vi "Align.vi"(6 "Variant in":variant, 7 "Shift Pressed?":bool, 8 "error in (no error)":errorcluster, 10 "QD Combo Box Ref":refnum<vi>, 11 "QD Launch VI Ref":refnum<vi>) -> (0 "error out":errorcluster, 4 "Variant out":variant)   [LabVIEW 2019]
doc: "Write a 1-2 sentence description of the functionality of your plugin here. Replace the \"$\" below with the character you wish to assign as the default shortcut for this plugin. Do not add any text after the 'Default Shortcut' line below.\n\nDefault Shortcut - [$]"
uses:
  <vilib>/Utility/traverseref.llb/TRef TravTarget.ctl
  <vilib>/Utility/traverseref.llb/VI Scripting - Traverse.lvlib
panel:
  in  "Undo Name":string="Quick Drop Keyboard Shortcut"
  # "Specify the name of the Undo transaction"
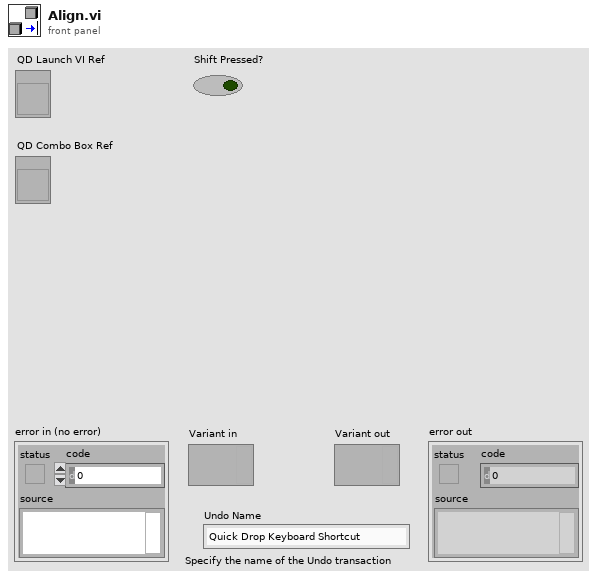
[diagram p1: front panel]
types:
  T1 = typedef "TRef TravTarget.ctl" = enum16{"FP", "BD", "Other"}
  T2 = enum32{"Top Edges", "Vertical Centers", "Bottom Edges", "Left Edges", "Horizontal Centers", "Right Edges"}
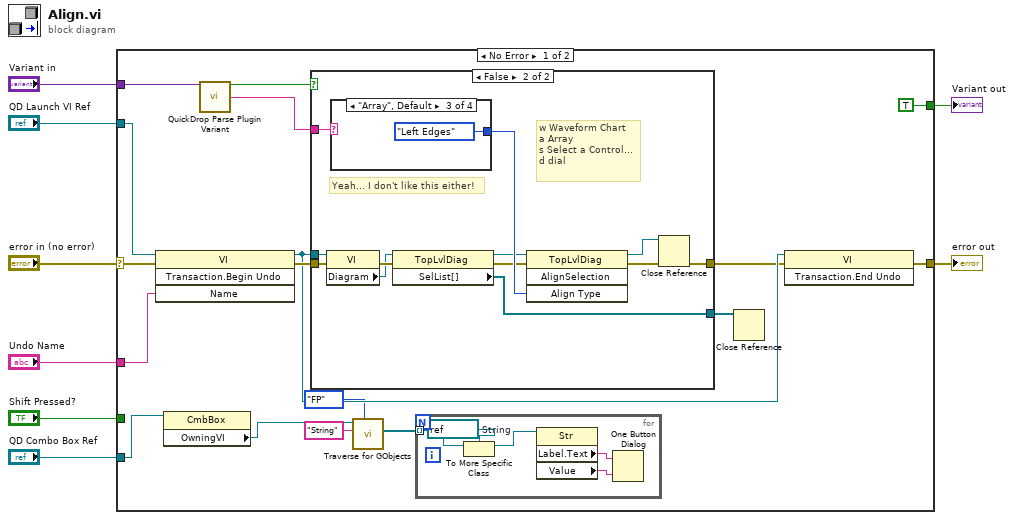
[diagram p0: block diagram]
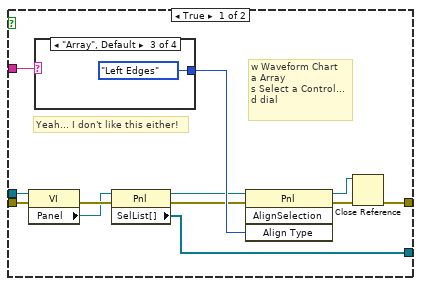
[diagram p2: hidden frame]
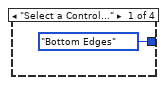
[diagram p3: hidden frame]
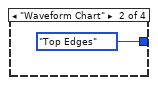
[diagram p4: hidden frame]
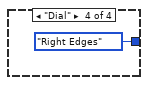
[diagram p5: hidden frame]
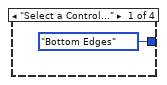
[diagram p6: hidden frame]
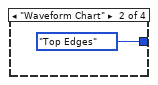
[diagram p7: hidden frame]
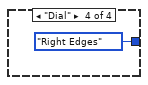
[diagram p8: hidden frame]
diagram:
  n1 = case shown="No Error" "error in (no error)" {
    selector: "error in (no error)" -> [w24 w63]
    tunnel: [w18 w63] -> w7
    tunnel: "QD Launch VI Ref" -> [w23 _]
    tunnel: "Shift Pressed?" -> [_ _]
    tunnel: "QD Combo Box Ref" -> [w13 _]
    tunnel: "Variant in" -> [w25 _]
    tunnel: "Undo Name" -> [w22 _]
    tunnel: [TRUE _] -> w1
    frame No Error {
      n2 = invoke class="VI" method="Transaction.Begin Undo"(reference=w23, error in=w24, "Name"=w22) -> (reference out=w17:refnum<vi>, error out=w19:errorcluster)  [unwired: 1 in, 2 out]
      n3 = property class="CmbBox"(reference=w13) -> ("OwningVI"=w12:refnum<vi>)  [unwired: 1 in, 2 out]
      n4 = call <vilib>:"QuickDrop Parse Plugin Variant.vi"("QDKS Variant in"=w25) -> ("QD Launch VI Panel?"=w20:bool, "Palette Object Name"=w16:string)  [unwired: 12 in, 1 out]
      n5 = case shown="False" w20 {
        tunnel: w19 -> [w42 w58]
        tunnel: w17 -> [w41 w57]
        tunnel: [w39 w47] -> w14
        tunnel: [w38 w55] -> w15
        tunnel: w16 -> [w35 w52]
        frame True {
          # "Yeah... I don't like this either!"
          # "w Waveform Chart\na Array\ns Select a Control...\nd dial"
          n6 = property class="VI"(reference=w41, error in=w42) -> (error out=w40:errorcluster, "Panel"=w37:refnum<vi>)  [unwired: 1 out]
          n7 = case shown="\"Array\", Default" w35 {
            tunnel: [T2."Bottom Edges" ("Align Type") T2."Top Edges" ("Align Type") T2."Left Edges" ("Align Type") T2."Right Edges" ("Align Type")] -> w36
            frame "Select a Control..." {
            }
            frame "Waveform Chart" {
            }
            frame "Array", Default {
            }
            frame "Dial" {
            }
          }
          n8 = property class="Pnl"(reference=w37, error in=w40) -> (reference out=w31:refnum<vi>, error out=w32:errorcluster, "SelList[]"=w38:refnum<vi>[])
          n9 = invoke class="Pnl" method="AlignSelection"(reference=w31, error in=w32, "Align Type"=w36) -> (reference out=w34:refnum<vi>, error out=w33:errorcluster)  [unwired: 1 in, 2 out]
          n10 = Close Reference(reference=w34, error in (no error)=w33) -> (error out=w39:errorcluster)
        }
        frame False {
          # "Yeah... I don't like this either!"
          # "w Waveform Chart\na Array\ns Select a Control...\nd dial"
          n11 = property class="VI"(reference=w57, error in=w58) -> (error out=w56:errorcluster, "Diagram"=w54:refnum<vi>)  [unwired: 1 out]
          n12 = case shown="\"Array\", Default" w52 {
            tunnel: [T2."Bottom Edges" ("Align Type") T2."Top Edges" ("Align Type") T2."Left Edges" ("Align Type") T2."Right Edges" ("Align Type")] -> w53
            frame "Select a Control..." {
            }
            frame "Waveform Chart" {
            }
            frame "Array", Default {
            }
            frame "Dial" {
            }
          }
          n13 = property class="TopLvlDiag"(reference=w54, error in=w56) -> (reference out=w51:refnum<vi>, error out=w50:errorcluster, "SelList[]"=w55:refnum<vi>[])
          n14 = invoke class="TopLvlDiag" method="AlignSelection"(reference=w51, error in=w50, "Align Type"=w53) -> (reference out=w48:refnum<vi>, error out=w49:errorcluster)  [unwired: 1 in, 2 out]
          n15 = Close Reference(reference=w48, error in (no error)=w49) -> (error out=w47:errorcluster)
        }
      }
      n16 = call <vilib>:"Traverse for GObjects.vi"("Traverse Target"=TRef_TravTarget."FP", "Class Name"="String", "VI Refnum"=w12) -> ("References"=w9:refnum<vi>[])  [unwired: 5 in, 3 out]
      n17 = for {
        tunnel: w9 -> [w30] mode=indexing
        w28 = refnum<vi> refnum  # String
        n18 = To More Specific Class(target class=w28, reference=w30) -> (specific class reference=w29:refnum<vi>)  [unwired: 1 in, 1 out]
        n19 = property class="Str"(reference=w29) -> ("Label.Text"=w26:string, "Value"=w27:string)  [unwired: 1 in, 2 out]
        n20 = One Button Dialog(message=w26, button name ("OK")=w27) -> ()  [unwired: 1 out]
      }
      n21 = Close Reference(reference=w15) -> ()  [unwired: 1 in, 1 out]
      n22 = invoke class="VI" method="Transaction.End Undo"(reference=w17, error in=w14) -> (error out=w18:errorcluster)  [unwired: 1 in, 2 out]
    }
    frame Error {
    }
  }
  "error out" <- w7
  "Variant out" <- w1
